vi "Get Order-RPM Spectral Map (DBL).vi"(6 "order range (auto)":T1 {"increment" format="%.2f"; "maximum" format="%.2f"; "minimum" format="%.2f"}, 7 "dB On (T)":bool=TRUE, 8 "error in (no error)":errorcluster, 9 "Gabor template":dbl[](array[numeric]) format="%.2f", 10 "sampling frequency [Hz]":dbl=1.0 format="%.2f", 11 "RefNum in":T2) -> (0 "error out":errorcluster, 1 "quantization info":cluster{"offset":dbl, "multiplier":dbl} {"multiplier" format="%.2f"; "offset" format="%.2f"}, 2 "spectral map":dbl[][](array[numeric]) format="%.2f", 3 "RefNum out":T2, 4 "order scale":cluster{"offset":dbl, "multiplier":dbl} {"multiplier" format="%.2f"; "offset" format="%.2f"}, 5 "rpm scale":cluster{"offset":dbl, "multiplier":dbl} {"multiplier" format="%.2f"; "offset" format="%.2f"})   [LabVIEW 2017, in "SoundVib_Gabor.lvlib"]
doc: "Generates an order-rpm spectral map of the data block referenced by <B>RefNum in</B>. You can use this polymorphic VI to return <B>spectral map</B> as a 2D array of double-precision, floating-point numbers or a 2D array of 8-bit unsigned integers. You must manually select the polymorphic instance to use. Use the DBL instance to obtain more accurate data. Use the U8 instance to reduce memory usage when the VI displays data."
uses:
  <vilib>/addons/Sound and Vibration/Order Analysis/Gabor Order Tracking/SoundVib_Gabor.lvlib
  <vilib>/addons/Sound and Vibration/Order Analysis/Ref Gabor Order Tracking/GT RefNum.ctl
  <resource>/sndvib.dll
panel:
  # "Get Order-RPM Spectral Map (DBL)"
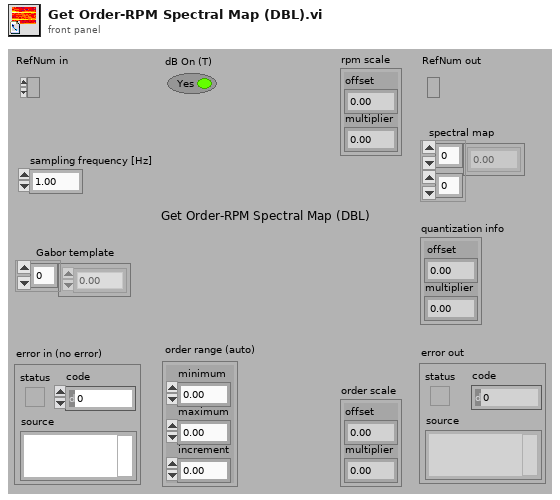
[diagram p1: front panel]
types:
  T1 = cluster{"minimum":dbl, "maximum":dbl, "increment":dbl}
  T2 = typedef "SoundVib_Gabor.lvlib/GT RefNum.ctl" = refnum<k1>
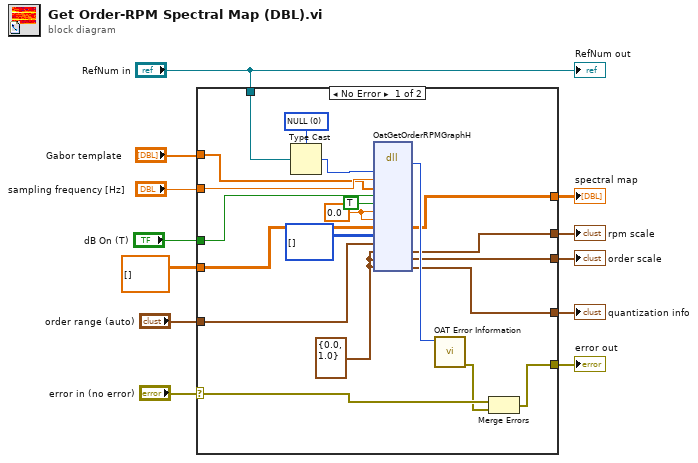
[diagram p0: block diagram]
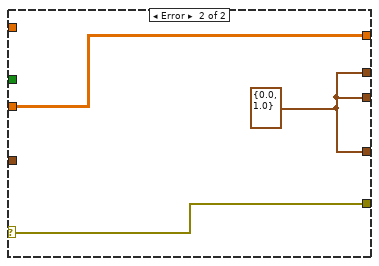
[diagram p2: hidden frame]
diagram:
  n1 = case shown="No Error" "error in (no error)" {
    selector: "error in (no error)" -> [w15 w35]
    tunnel: [w13 w35] -> w2
    tunnel: "RefNum in" -> [w31 _]
    tunnel: [w18 w34] -> w4
    tunnel: [w23 w33] -> w9
    tunnel: [w19 w34] -> w6
    tunnel: [w20 w34] -> w5
    tunnel: "sampling frequency [Hz]" -> [w29 _]
    tunnel: "dB On (T)" -> [w26 _]
    tunnel: "Gabor template" -> [w28 _]
    tunnel: "order range (auto)" -> [w22 _]
    tunnel: dbl[][] [] ("Graph") -> [w16 w33]
    frame No Error {
      w21 = cluster{"Z Min":dbl, "Z Step":dbl} {"Z Min"=0.0, "Z Step"=1.0}
      w24 = 0.0 ("uCutRatio")
      w32 = u32 0 items=["NULL"]
      n2 = Type Cast(type=w32, x=w31) -> (*(type *) &x=w30:u32)
      n3 = dll-call lib="C:/Program Files (x86)/National Instruments/LabVIEW 2017/resource/sndvib.*" fn="OatGetOrderRPMGraphH"("Ref In"=w30, "fs"=w29, "CntFreq"=w28, "bLogZ"=w26, "bGetDBL"=TRUE ("dB On (T)"), "uCutRatio"=w24, "dCutRatio"=w24, "DBLGraph"=w16, "U8Graph"=u8[][] [] ("Graph"), "OrderRange"=w22, "XScale"=w21, "YScale"=w21, "ZScale"=w21) -> ("return type"=w27:i32, "DBLGraph"=w23:dbl[][], "XScale"=w20:cluster{"Z Min":dbl, "Z Step":dbl}, "YScale"=w19:cluster{"Z Min":dbl, "Z Step":dbl}, "ZScale"=w18:cluster{"Z Min":dbl, "Z Step":dbl})  [unwired: 12 in, 2 out]
      n4 = call <vilib>:"OAT Error Information.vi"("error code"=w27) -> ("error out"=w14:errorcluster)  [unwired: 6 in]
      n5 = Merge Errors(w15, w14) -> (w13:errorcluster)
    }
    frame Error {
      w34 = cluster{"Z Min":dbl, "Z Step":dbl} {"Z Min"=0.0, "Z Step"=1.0}
    }
  }
  "error out" <- w2
  "quantization info" <- w4
  "order scale" <- w6
  "rpm scale" <- w5
  "spectral map" <- w9
  "RefNum out" <- "RefNum in"
